vi "Teleop.vi"(10 "Match Info":T1={"Autonomous Elapsed Seconds"=0.0, "TeleOp Elapsed Seconds"=0.0, "Disabled Elapsed Seconds"=0.0, "Visited Autonomous"=FALSE, "Visited TeleOp"=FALSE, "Visited Disabled"=FALSE, "Autonomous Settings"={"Autonomous Style"=enum."Independent", "VI Refnum"=refnum}}, 11 "Call Context":T2) -> ()   [LabVIEW 2018]
doc: "This VI is called for each enabled TeleOp packet received from the DS. It is typically used to read from joysticks and other inputs and update I/O or setpoints for timed control loops. It should complete and return within 20 milliseconds or risk missing DS packets."
uses:
  <vilib>/Rock Robotics/WPI/DriverStation/WPI_DriverStationDerivedRobotMode.ctl
  <vilib>/Rock Robotics/WPI/DriverStation/WPI_DriverStationMatch Info.ctl
  Logging/DataNames.ctl
  <vilib>/Rock Robotics/WPI/Utilities/WPI_GetSetVariantRefNum.vi
  <vilib>/Rock Robotics/Network Tables/NT Write Number.vi
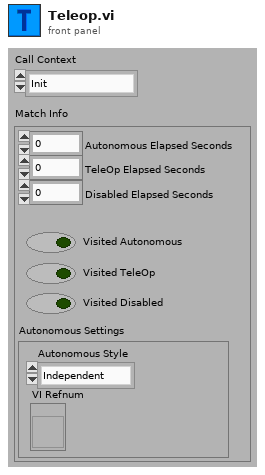
[diagram p1: front panel]
types:
  T1 = typedef "WPI_DriverStationMatch Info.ctl" = cluster{"Autonomous Elapsed Seconds":dbl, "TeleOp Elapsed Seconds":dbl, "Disabled Elapsed Seconds":dbl, "Visited Autonomous":bool, "Visited TeleOp":bool, "Visited Disabled":bool, "Autonomous Settings":cluster{"Autonomous Style":enum16{"Iterative", "Independent"}, "VI Refnum":refnum<vi>}}
  T2 = typedef "WPI_DriverStationDerivedRobotMode.ctl" = enum16{"Init", "Execute", "Stop"}
  T3 = typedef "DataNames.ctl" = enum16{"RobotMode", "FMSConnected", "DriveLeft", "DriveRight", "FloorHatchIntakeMotor", "SolenoidDirection", "EncoderLeft", "EncoderRight", "ArmEncoder", "ArmTopLimitSwitch", "ArmBottomLimitSwitch", "HatchLimitSwitch", "Yaw", "CheesyStraightJoystick", "CheesyTurnJoystick", "XCoordinate", "YCoordinate", "CPU", "DriveOperation", "Battery"}
  T4 = typedef "WPI_JoystickDevRef.ctl" = cluster{"Device":T5}
  T5 = typedef "WPI_JoystickDeviceEnum.ctl" = enum16{"USB 0", "USB 1", "USB 2", "USB 3", "USB 4", "USB 5"}
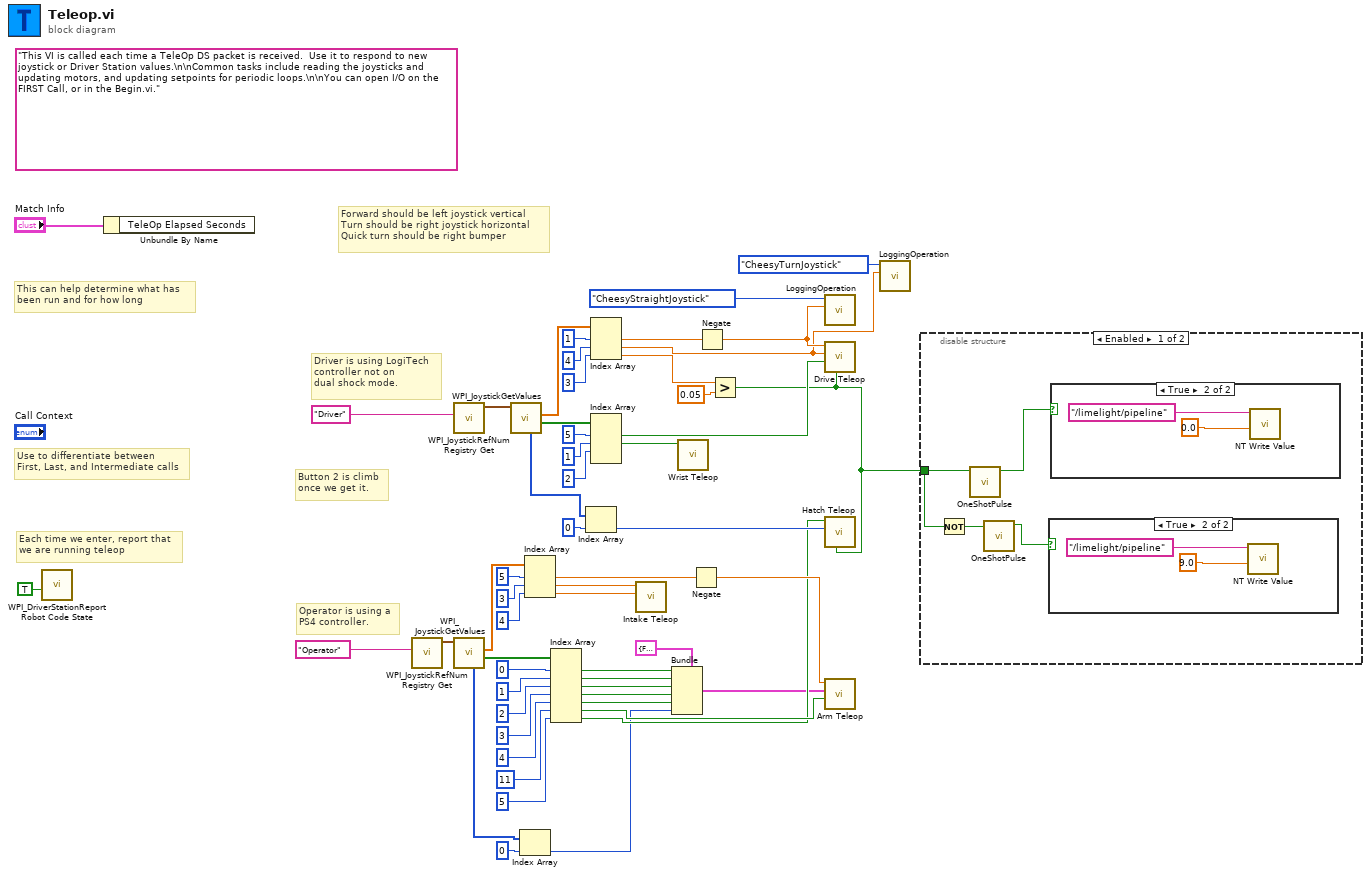
[diagram p0: block diagram]
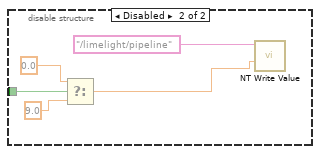
[diagram p4: hidden frame]
diagram:
  (unwired) "This VI is called each time a TeleOp DS packet is received.  Use it to respond to new joystick or Driver Station values.\n\nCommon tasks include reading the joysticks and updating motors, and updating setpoints for periodic loops.\n\nYou can open I/O on the FIRST Call, or in the Begin.vi."
  # "Driver is using LogiTech\ncontroller not on\ndual shock mode."
  # "Button 2 is climb\nonce we get it."
  # "Operator is using a\nPS4 controller."
  # "Forward should be left joystick vertical\nTurn should be right joystick horizontal\nQuick turn should be right bumper"
  # "Each time we enter, report that\nwe are running teleop"
  # "Use to differentiate between\nFirst, Last, and Intermediate calls"
  # "This can help determine what has\nbeen run and for how long"
  n1 = call <vilib>:"WPI_DriverStationReport Robot Code State.vi"("TeleOp"=TRUE ("Autonomous")) -> ()  [unwired: 10 in, 1 out]
  n2 = Unbundle By Name("Match Info") -> ()  [unwired: 1 out]
  n3 = call <vilib>:"WPI_JoystickRefNum Registry Get.vi"("refnum name"="Operator") -> ("JoystickDevRef"=w50:T4)  [unwired: 1 in, 9 out]
  n4 = call <vilib>:"WPI_JoystickRefNum Registry Get.vi"("refnum name"="Driver") -> ("JoystickDevRef"=w52:T4)  [unwired: 1 in, 9 out]
  n5 = call <vilib>:"WPI_JoystickGetValues.vi"("JoystickDevRef"=w50) -> ("Buttons"=w21:bool[], "Axes"=w49:dbl[], "POVs"=w20:i16[])  [unwired: 6 in, 2 out]
  n6 = call <vilib>:"WPI_JoystickGetValues.vi"("JoystickDevRef"=w52) -> ("Buttons"=w34:bool[], "Axes"=w33:dbl[], "POVs"=w40:i16[])  [unwired: 6 in, 2 out]
  n7 = Index Array(array=w20, index=0) -> (element=w11:i16)
  n8 = Index Array(array=w49, index #1=5 ("index"), index #2=3 ("index"), index #3=4 ("index")) -> (element #1=w46:dbl, element #2=w42:dbl, element #3=w41:dbl)
  n9 = Index Array(array=w21, index #1=0 ("index"), index #2=1 ("index"), index #3=2 ("index"), index #4=3 ("index"), index #5=4 ("index"), index #6=11 ("index"), index #7=5 ("index")) -> (element #1=w28:bool, element #2=w27:bool, element #3=w26:bool, element #4=w25:bool, element #5=w24:bool, element #6=w23:bool, element #7=w22:bool)
  n10 = Index Array(array=w40, index=0) -> (element=w43:i16)
  n11 = Index Array(array=w33, index #1=1 ("index"), index #2=4 ("index"), index #3=3 ("index")) -> (element #1=w36:dbl, element #2=w3:dbl, element #3=w35:dbl)
  n12 = Index Array(array=w34, index #1=5 ("index"), index #2=1 ("index"), index #3=2 ("index")) -> (element #1=w8:bool, element #2=w7:bool)  [unwired: 1 in, 2 out]
  n13 = call "Intake Teleop.vi"("Right Trigger"=w41, "Left Trigger"=w42) -> ()  [unwired: 10 in]
  n14 = Bundle(cluster=cluster{bool, bool, bool, bool, bool, i32} {FALSE, FALSE, FALSE, FALSE, FALSE, 0}, w28, w27, w26, w25, w24, w11) -> (w12:cluster{bool, bool, bool, bool, bool, i32})
  n15 = call "Wrist Teleop.vi"("Wrist Toggle"=w7) -> ()  [unwired: 11 in]
  n16 = Negate(x=w46) -> (-x=w45:dbl)
  n17 = Negate(x=w36) -> (-x=w47:dbl)
  n18 = Greater?(x=w35, y=0.05) -> (0:w1:bool)
  n19 = call "LoggingOperation.vi"("Data"=w47, "Name"=DataNames."CheesyStraightJoystick") -> ()  [unwired: 9 in, 1 out]
  n20 = call "Drive Teleop.vi"("Auto Align"=w1, "Quick turn"=w8, "Turn"=w3, "Forward"=w47) -> ()  [unwired: 8 in]
  n21 = call "Hatch Teleop.vi"("Auto Align"=w1, "POV Value"=w43, "Hatch toggle"=w22) -> ()  [unwired: 9 in]
  n22 = call "Arm Teleop.vi"("Slow Lift?"=w23, "Height Presets"=w12, "Speed"=w45) -> ()  [unwired: 9 in]
  n23 = call "LoggingOperation.vi"("Data"=w3, "Name"=DataNames."CheesyTurnJoystick") -> ()  [unwired: 9 in, 1 out]
  n24 = disable-structure shown="Enabled" {
    disable-tunnel: w1 -> [w58 w67]
    frame Enabled {
      n25 = Not(x=w58) -> (.not. x?=w57:bool)
      n26 = call "OneShotPulse.vi"("Input"=w58) -> ("Output"=w59:bool)  [unwired: 10 in]
      n27 = call "OneShotPulse.vi"("Input"=w57) -> ("Output"=w56:bool)  [unwired: 10 in]
      n28 = case shown="True" w56 {
        frame False {
        }
        frame True {
          n29 = call-poly <vilib>:"NT Write Value.vi"("Numeric"=9.0, "Name"="/limelight/pipeline") -> ()  [unwired: 9 in, 1 out]
        }
      }
      n30 = case shown="True" w59 {
        frame False {
        }
        frame True {
          n31 = call-poly <vilib>:"NT Write Value.vi"("Numeric"=0.0, "Name"="/limelight/pipeline") -> ()  [unwired: 9 in, 1 out]
        }
      }
    }
    frame Disabled {
      n32 = Select(t=0.0 ("Numeric"), s=w67, f=9.0 ("Numeric")) -> (s? t:f=w64:dbl)
      n33 = call-poly <vilib>:"NT Write Value.vi"("Numeric"=w64, "Name"="/limelight/pipeline") -> ()  [unwired: 9 in, 1 out]
    }
  }
